vi "Simple Radar Plot.vi"() -> ()   [LabVIEW 2023]
doc: "Uses the Radar Plot VI to draw a radar plot in a picture indicator."
panel:
  in  "Data":string[][](table)=[["1", "33", "4", "3", "2", "3"], ["4", "26", "12", "8", "3", "2"], ["2", "12", "2", "14", "4", "3"], ["3", "44", "8", "12", "9", "12"]]
  out "Radar Plot":picture
  # "Overview: Uses the Radar Plot VI to draw a radar plot in a picture indicator.\nInstructions:\nRun the VI."
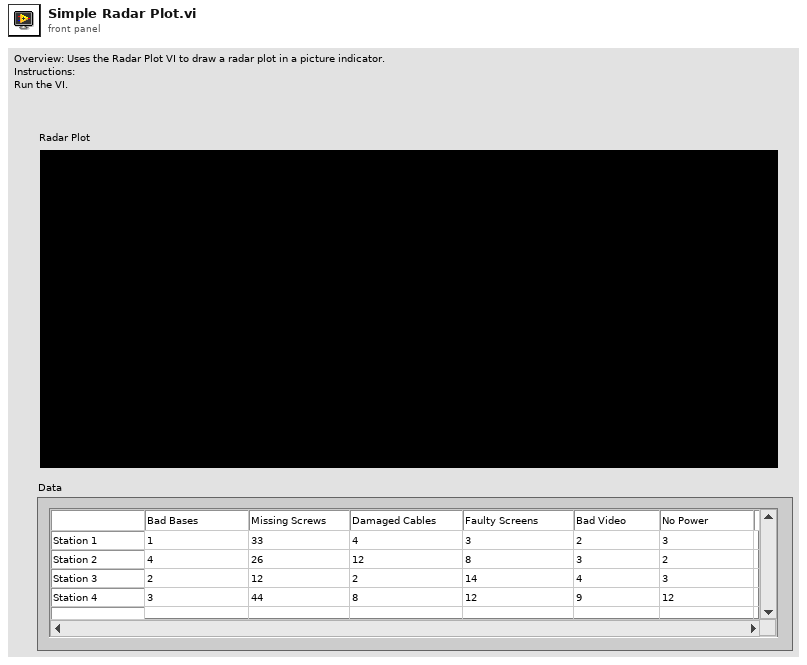
[diagram p1: front panel]
types:
  T1 = cluster{"Legend Position":u16, "Legend Text Color":u32}
  T2 = typedef "LVBoundsTypeDef.ctl" = cluster{"Width":u32, "Height":u32}
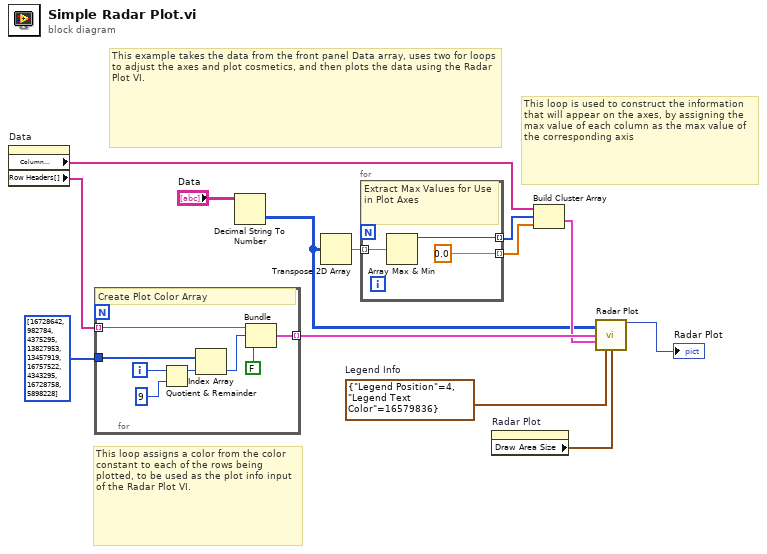
[diagram p0: block diagram]
diagram:
  w2 = T1 {"Legend Position"=4, "Legend Text Color"=16579836}  # Legend Info
  # "This loop is used to construct the information that will appear on the axes, by assigning the max value of each column as the max value of the corresponding axis"
  # "This loop assigns a color from the color constant to each of the rows being plotted, to be used as the plot info input of the Radar Plot VI."
  # "This example takes the data from the front panel Data array, uses two for loops to adjust the axes and plot cosmetics, and then plots the data using the Radar Plot VI."
  n1 = property on="Data" class="Tbl (strict)"() -> ("Column Headers[]"=w4:string[], "Row Headers[]"=w5:string[])  [unwired: 2 in, 2 out]
  n2 = for {
    tunnel: u32[] [16728642, 982784, 4375295, 13827953, 13457919, 16757522, 4343295, 16728758, 5898228] ("Array") -> [w20]
    tunnel: [w18] -> w12 mode=indexing
    tunnel: w5 -> [w15] mode=indexing
    i -> [w17]
    # "Create Plot Color Array"
    n3 = Quotient & Remainder(x=w17, y=9) -> (x-y*floor(x/y)=w21:i32)  [unwired: 1 out]
    n4 = Index Array(array=w20, index=w21) -> (element=w19:u32)
    n5 = Bundle(w15, "Plot.Plot Color"=w19, FALSE) -> (w18:cluster{string, "Plot.Plot Color":u32, bool})  [unwired: 1 in]
  }
  n6 = Decimal String To Number(string="Data") -> (number=w1:i32[][])  [unwired: 2 in, 1 out]
  n7 = Transpose 2D Array(2D array=w1) -> (transposed array=w6:i32[][])
  n8 = for {
    tunnel: w6 -> [w24] mode=indexing
    tunnel: [w23] -> w9 mode=indexing
    tunnel: [0.0] -> w8 mode=indexing
    # "Extract Max Values for Use in Plot Axes"
    n9 = Array Max & Min(array=w24) -> (max value=w23:i32)  [unwired: 3 out]
  }
  n10 = property on="Radar Plot" class="Pict"() -> ("Draw Area Size"=w10:T2)  [unwired: 2 in, 2 out]
  n11 = Build Cluster Array(w4, w9, w8) -> (w7:cluster{string, i32, dbl}[])
  n12 = call <vilib>:"Radar Plot.vi"("data"=w1, "plot info"=w12, "axis info"=w7, "legend info"=w2, "dimension (w,h)"=w10) -> ("new picture"=→"Radar Plot":picture)  [unwired: 10 in]
